vi "RANGE General Factors.vi"(8 "Error In":errorcluster, 11 "Gas Type String":string) -> (0 "Error Out":errorcluster, 2 "Flow Rate Factor":dbl)   [LabVIEW 2023]
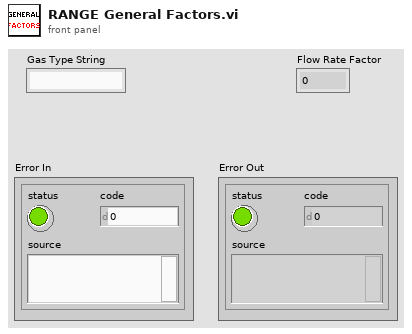
[diagram p1: front panel]
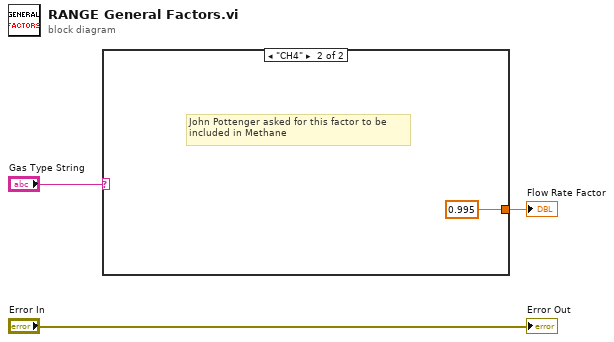
[diagram p0: block diagram]
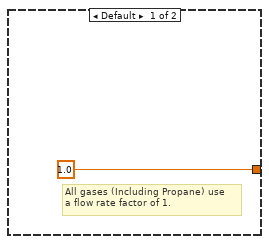
[diagram p2: hidden frame]
diagram:
  n1 = case shown="\"CH4\"" "Gas Type String" {
    tunnel: [1.0 0.995] -> w3
    frame Default {
      # "All gases (Including Propane) use\na flow rate factor of 1."
    }
    frame "CH4" {
      # "John Pottenger asked for this factor to be \nincluded in Methane"
    }
  }
  "Flow Rate Factor" <- w3
  "Error Out" <- "Error In"
